vi "_FPGA System Polling.vi"(4 "error in (no error)":errorcluster, 5 "Waiting (F)":bool, 6 "Connected?":bool, 7 "CurInstrState":T3, 8 "High Vac Reached?":bool) -> (1 "Running":bool, 3 "Next InstrState":T3)   [LabVIEW 2018]
uses:
  Type/_RT Instrument State.ctl
  Type/_RT Polling Settings.ctl
  Type/_LCD Line2 Msg.ctl
  Type/_LED States.ctl
  Type/_LCD Line1 Msg.ctl
  Type/_RW Status.ctl
  Type/_Pump Parameter.ctl
  _RT Global.vi
  <vilib>/Utility/error.llb/Error Cluster From Error Code.vi
  <vilib>/rvi/errors/niLvFpgaAdjustHostInterfaceError.vi
  <vilib>/rvi/interface/nirviReadWriteControl/nirviReadWriteControl.xnode
  Type/FPGA Typedef.ctl
  FPGA Bitfiles/FPGA9607.lvbitx
  NiFpgaLv.dll
panel:
  out "Raw Reading":sgl
  in  "Polling Settings":T1[](array[typedef])=[{"ADC Ch"=119, "UserVal"=FALSE, "LowVal"=0.0, "HighVal"=89.0, "Fail Level"=50, "Err"="VG Disconnected/Broken Warning", "Line2Msg"=13, "InstrState"=enum."Ready", "Code"="004"}, {"ADC Ch"=119, "UserVal"=FALSE, "LowVal"=255.0, "HighVal"=300.0, "Fail Level"=50, "Err"="VG Disconnected/Broken Warning", "Line2Msg"=13, "InstrState"=enum."Ready", "Code"="004"}, {"ADC Ch"=119, "UserVal"=FALSE, "LowVal"=150.0, "HighVal"=254.0, "Fail Level"=50, "Err"="Overpressure Warning", "Line2Msg"=13, "InstrState"=enum."Ready", "Code"="006"}, {"ADC Ch"=64, "UserVal"=FALSE, "LowVal"=-5.0, "HighVal"=0.249, "Fail Level"=39, "Err"="Drying Gas Low", "Line2Msg"=4, "InstrState"=enum."Turbopump Ready", "Code"=""}, {"ADC Ch"=74, "UserVal"=FALSE, "LowVal"=0.36, "HighVal"=5.0, "Fail Level"=10, "Err"="Foreline Pressure Failure", "Line2Msg"=2, "InstrState"=enum."Fault", "Code"="001"}, {"ADC Ch"=25, "UserVal"=TRUE, "LowVal"=91.0, "HighVal"=200.0, "Fail Level"=35, "Err"="Q2 Board Slot 5 Overheating", "Line2Msg"=5, "InstrState"=enum."Turbopump Ready-Waiting", "Code"="008"}, {"ADC Ch"=49, "UserVal"=TRUE, "LowVal"=91.0, "HighVal"=200.0, "Fail Level"=35, "Err"="Q1 Board Slot 9 Overheating", "Line2Msg"=5, "InstrState"=enum."Turbopump Ready-Waiting", "Code"="009"}, {"ADC Ch"=57, "UserVal"=TRUE, "LowVal"=91.0, "HighVal"=200.0, "Fail Level"=35, "Err"="M1RF Board Slot 13 Overheating", "Line2Msg"=5, "InstrState"=enum."Turbopump Ready-Waiting", "Code"="010"}, {"ADC Ch"=26, "UserVal"=TRUE, "LowVal"=91.0, "HighVal"=200.0, "Fail Level"=35, "Err"="Q2 Board Slot 5 Overheating", "Line2Msg"=5, "InstrState"=enum."Turbopump Ready-Waiting", "Code"="008"}, {"ADC Ch"=50, "UserVal"=TRUE, "LowVal"=91.0, "HighVal"=200.0, "Fail Level"=35, "Err"="Q1 Board Slot 9 Overheating", "Line2Msg"=5, "InstrState"=enum."Turbopump Ready-Waiting", "Code"="009"}, {"ADC Ch"=58, "UserVal"=TRUE, "LowVal"=91.0, "HighVal"=200.0, "Fail Level"=35, "Err"="M1RF Board Slot 13 Overheating", "Line2Msg"=5, "InstrState"=enum."Turbopump Ready-Waiting", "Code"="010"}, {"ADC Ch"=113, "UserVal"=FALSE, "LowVal"=1.0, "HighVal"=2.0, "Fail Level"=40, "Err"="Source 1 Interlock Activated", "Line2Msg"=6, "InstrState"=enum."Source Standby", "Code"=""}, {"ADC Ch"=114, "UserVal"=FALSE, "LowVal"=1.0, "HighVal"=2.0, "Fail Level"=40, "Err"="Source 2 Interlock Activated", "Line2Msg"=7, "InstrState"=enum."Source Standby", "Code"=""}, {"ADC Ch"=14, "UserVal"=FALSE, "LowVal"=4.5, "HighVal"=10.0, "Fail Level"=35, "Err"="Heater PS Current High", "Line2Msg"=8, "InstrState"=enum."Turbopump Ready-Waiting", "Code"="011"}, {"ADC Ch"=51, "UserVal"=TRUE, "LowVal"=-9999.0, "HighVal"=-12.0, "Fail Level"=35, "Err"="Q1 Tuning Error", "Line2Msg"=5, "InstrState"=enum."Turbopump Ready-Waiting", "Code"="012"}, {"ADC Ch"=27, "UserVal"=TRUE, "LowVal"=-9999.0, "HighVal"=-12.0, "Fail Level"=35, "Err"="Q2 Tuning Error", "Line2Msg"=5, "InstrState"=enum."Turbopump Ready-Waiting", "Code"="013"}, {"ADC Ch"=59, "UserVal"=TRUE, "LowVal"=-9999.0, "HighVal"=-12.0, "Fail Level"=35, "Err"="M1 Tuning Error", "Line2Msg"=5, "InstrState"=enum."Turbopump Ready-Waiting", "Code"="014"}, {"ADC Ch"=120, "UserVal"=FALSE, "LowVal"=0.0, "HighVal"=0.0, "Fail Level"=32, "Err"="Card Cage Door Interlock Activated", "Line2Msg"=9, "InstrState"=enum."Go to 24V Standby", "Code"=""}, {"ADC Ch"=121, "UserVal"=FALSE, "LowVal"=0.0, "HighVal"=0.0, "Fail Level"=35, "Err"="Vacuum Ready Tripped", "Line2Msg"=2, "InstrState"=enum."Turbopump Ready-Waiting", "Code"="015"}, {"ADC Ch"=76, "UserVal"=FALSE, "LowVal"=0.0, "HighVal"=2.5, "Fail Level"=39, "Err"="Drying Gas Supply Low", "Line2Msg"=4, "InstrState"=enum."Turbopump Ready", "Code"=""}, {"ADC Ch"=78, "UserVal"=FALSE, "LowVal"=0.0, "HighVal"=3.5, "Fail Level"=39, "Err"="Source Gas Supply Low", "Line2Msg"=12, "InstrState"=enum."Turbopump Ready", "Code"=""}, {"ADC Ch"=100, "UserVal"=FALSE, "LowVal"=0.0, "HighVal"=0.0, "Fail Level"=32, "Err"="Electronics is off", "Line2Msg"=5, "InstrState"=enum."Go to 24V Standby", "Code"="017"}, {"ADC Ch"=72, "UserVal"=FALSE, "LowVal"=-1.0, "HighVal"=0.3, "Fail Level"=49, "Err"="Exhaust Gas Low", "Line2Msg"=15, "InstrState"=enum."Ready", "Code"=""}, {"ADC Ch"=81, "UserVal"=TRUE, "LowVal"=26.0, "HighVal"=30.0, "Fail Level"=50, "Err"="RF Board Power Supply Error", "Line2Msg"=0, "InstrState"=enum."Ready", "Code"=""}, {"ADC Ch"=82, "UserVal"=TRUE, "LowVal"=-30.0, "HighVal"=-26.0, "Fail Level"=50, "Err"="RF Board Power Supply Error", "Line2Msg"=0, "InstrState"=enum."Ready", "Code"=""}, {"ADC Ch"=83, "UserVal"=TRUE, "LowVal"=45.0, "HighVal"=65.0, "Fail Level"=50, "Err"="Heater Power Supply Error", "Line2Msg"=0, "InstrState"=enum."Ready", "Code"=""}, {"ADC Ch"=85, "UserVal"=TRUE, "LowVal"=22.0, "HighVal"=26.0, "Fail Level"=50, "Err"="24 V Mains Power Supply Error", "Line2Msg"=0, "InstrState"=enum."Ready", "Code"=""}, {"ADC Ch"=86, "UserVal"=TRUE, "LowVal"=13.0, "HighVal"=16.0, "Fail Level"=50, "Err"="ADC/Board Power Supply Error", "Line2Msg"=0, "InstrState"=enum."Ready", "Code"=""}, {"ADC Ch"=87, "UserVal"=TRUE, "LowVal"=-16.0, "HighVal"=-13.0, "Fail Level"=50, "Err"="ADC/Board Power Supply Error", "Line2Msg"=0, "InstrState"=enum."Ready", "Code"=""}] {"Line2Msg" items=["Same", "Empty", "VacFail", "Cancel", "CheckGas", "EleFail", "Probe1Fail", "Probe2Fail", "HeaterFail", "DoorOpen", "CheckComm", "PressStart", "CheckSource", "VacWarn", "ForelineHigh", "SourceExhaustLow"]}
  # "0   119  50 vacuum gauge disconnected\n1   119  50 vacuum gauge disconnected\n2   119  50 overpressure warning\n3   64    39 drying gas low\n4   74    10 foreline pressure failure\n5   25    35 Q2 board slot 5 overheating\n6   49    35 Q1 board slot 9 overheating\n7   57    35 M1RF board slot 13 overheating\n8   26    35 Q2 board slot 5 overheating\n9   50    35 Q1 board slot 9 overheating\n10  58    35 M1RF board slot 13 overheating\n11 113  40 source 1 interlock activated\n12 114  40 source 2 interlock activated\n13  14    35 heater PS currect high\n14  51    35 Q1 tuning error\n15  27    35 Q2 tuning error\n16  59    35 M1 tuning error\n17 120  32 card cage door interlock activated\n18 121  35 vacuum ready tripped\n19  76    40 drying gas supply low\n20  78    40 source gas supply low\n21 100  32 electronics is off\n22  72    50 exhaust gas low\n23  81    50 RF board power supply error\n24  82    50 RF board power supply error\n25  83    50 heater power supply error\n26  85    50 24 V mains power supply error\n27  86    50 ADC/board power supply error\n28  87    50 ADC/board power supply error"
  # "same"
  # "4.6 -> 5.1"
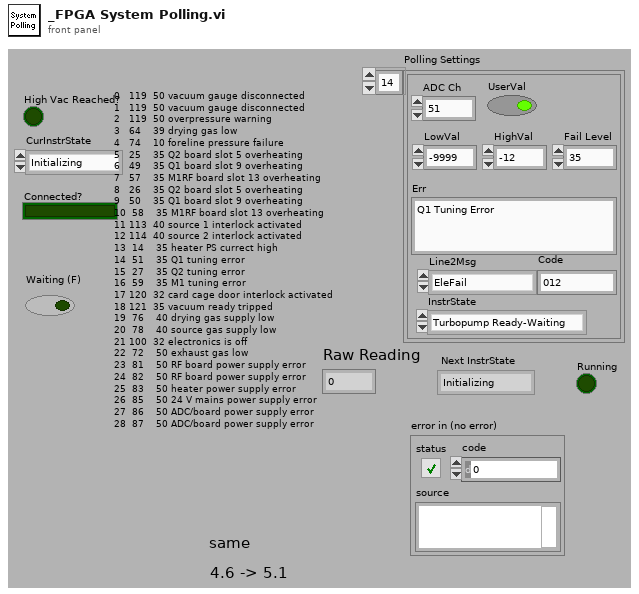
[diagram p1: front panel]
types:
  T1 = typedef "_RT Polling Settings.ctl" = cluster{"ADC Ch":u8, "UserVal":bool, "LowVal":sgl, "HighVal":sgl, "Fail Level":u8, "Err":string, "Line2Msg":T2, "InstrState":T3, "Code":string}
  T2 = typedef "_LCD Line2 Msg.ctl" = u16
  T3 = typedef "_RT Instrument State.ctl" = enum16{"Initializing", "Mass Spectrometer is Off", "Starting Up", "Turning Power Off", "Going to Standby", "Roughing Pump Ready", "Turning Turbo Off", "Turbo Startup", "Turbopump Ready", "Checking Vacuum", "Going to Ready", "Ready", "Running", "Source Standby", "Lost Communication", "Shutting Down", "Fault", "24V Standby", "Go to 24V Standby", "Turbopump Ready-Waiting"}
  T4 = typedef "_RT Startup Options.ctl" = cluster{"Door":bool, "Curtain":bool, "Pressure":bool, "Turbo":bool, "SysPoll":bool, "GasFlag":bool, "SourceExhaust":bool}
  T5 = typedef "_LED States.ctl" = enum8{"Idle", "Solid B", "Solid R", "Solid P", "Off B", "Off R", "Off P", "Off BRP", "Off RP", "Flash R&P", "Flash P"}
  T6 = typedef "_Pump Parameter.ctl" = enum16{"Turn Pump Motor On", "Turn Pump Motor Off", "Read Pump Oil Deficiency", "Read Rotation Switch Point Attained", "Read Ele. Drive Over Temperature", "Read Pump Over Temperature", "Read Set Rotation Speed Attained", "Read Turbopump Accelerates", "Read Actual Rotation Speed in Hz", "Read Motor Current in A", "Read Operating Hours in h", "Read Motor Voltage in V", "Read Motor Power in W", "Set Rotation Speed Switchpoint in %", "Clear Error", "Read Error Code", "Read Bearing Temperature", "Read Hardware Version", "Read Firmware Version", "Read Operating Hours (Drive)", "Read Rotational Speed (rpm)", "Read Power Stage Temperature", "Read Electronics Temperature", "Read Upper Pump Temperature", "Read Motor Temperature", "Read Error Code History, 1", "Read Error Code History, 2", "Read Error Code History, 3", "Read Error Code History, 4", "Read Error Code History, 5", "Read Error Code History, 6", "Read Error Code History, 7", "Read Error Code History, 8", "Read Error Code History, 9", "Read Error Code History, 10"}
  T7 = typedef "_RW Status.ctl" = enum8{"Done", "Do Read", "Do Write", "Set Latch1", "Set Latch2", "Set Latch3", "Set Latch4", "RP ON", "EL ON", "Serial Send", "Set LC Out", "Get LC In", "Read VAC", "Table Test", "Get Interlock", "Do Read2", "Do Write2"}
  T8 = typedef "FPGA Typedef.ctl" = refnum<k20>
  T9 = typedef "_LCD Line1 Msg.ctl" = u16
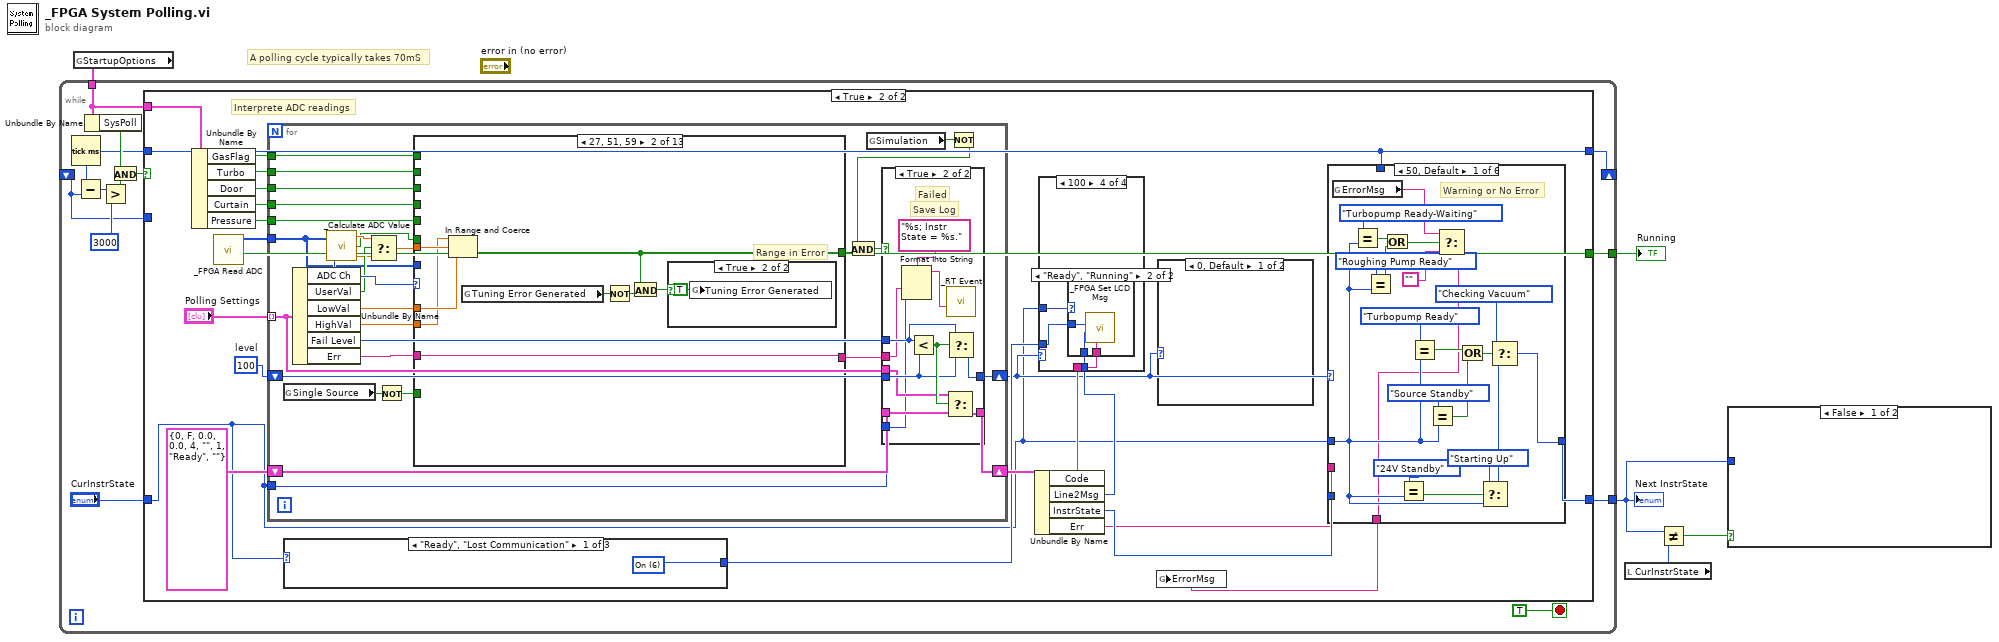
[diagram p0: block diagram]
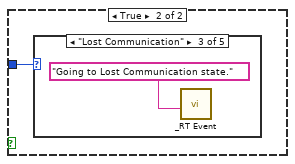
[diagram p2: hidden frame]
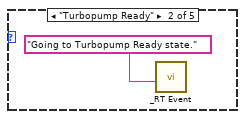
[diagram p4: hidden frame]
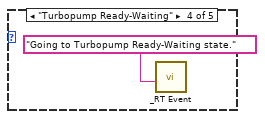
[diagram p5: hidden frame]
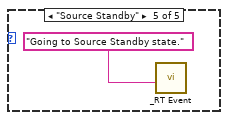
[diagram p6: hidden frame]
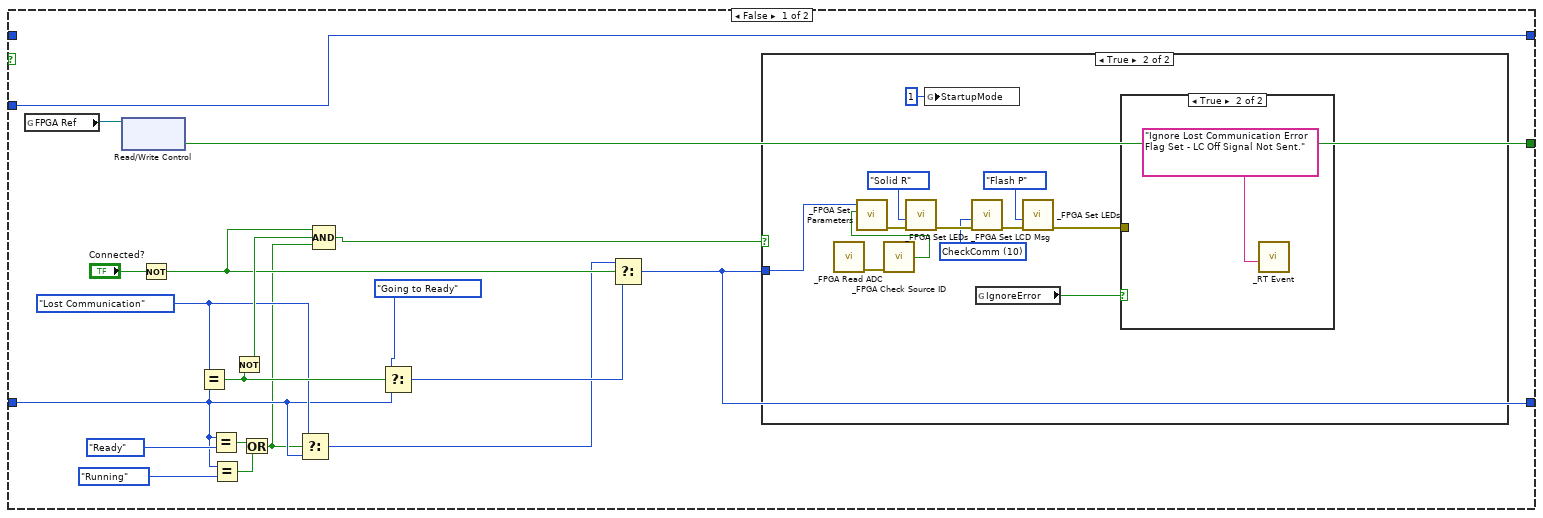
[diagram p7: hidden frame]
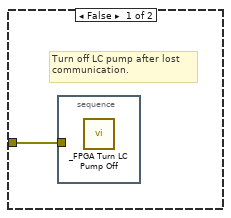
[diagram p9: hidden frame]
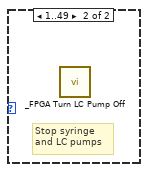
[diagram p10: hidden frame]
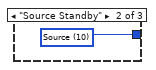
[diagram p11: hidden frame]
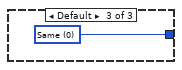
[diagram p12: hidden frame]
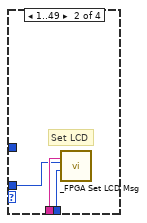
[diagram p14: hidden frame]
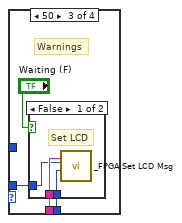
[diagram p15: hidden frame]
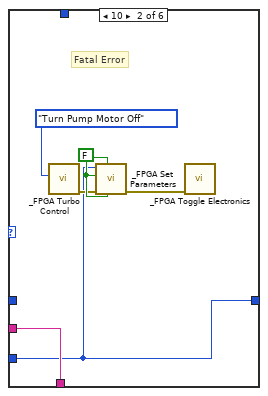
[diagram p18: hidden frame]
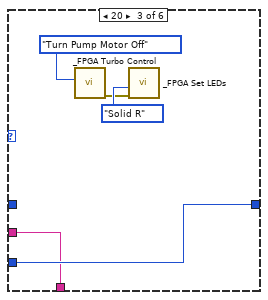
[diagram p19: hidden frame]
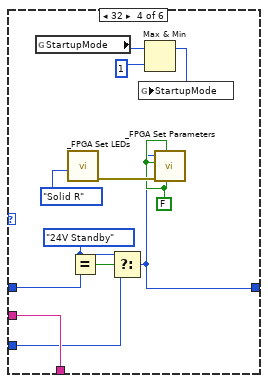
[diagram p20: hidden frame]
diagram:
  # "A polling cycle typically takes 70mS"
  n1 = global read "_RT Global.vi" "StartupOptions"() -> (w4:T4)
  n2 = while {
    tunnel: [w16] -> w1
    shift-right: [w7] -> _
    shift-left: _ -> [w6]
    tunnel: [w13] -> w5
    tunnel: w4 -> [w9]
    stop <- TRUE stop-if-true
    n3 = Tick Count (ms)() -> (millisecond timer value=w8:u32)
    n4 = Subtract(x=w8, y=w6) -> (x-y=w15:u32)
    n5 = Unbundle By Name(w9) -> ("SysPoll"=w12:bool)
    n6 = Greater?(x=w15, y=3000) -> (0:w11:bool)
    n7 = And(x=w12, y=w11) -> (x .and. y?=w10:bool)
    n8 = case shown="True" w10 {
      tunnel: [w19 w70] -> w16
      tunnel: "CurInstrState" -> [w24 w52]
      tunnel: [w30 w73] -> w13
      tunnel: w9 -> [_ w68]
      tunnel: w8 -> [_ w53]
      tunnel: [w33 w53] -> w7
      tunnel: w6 -> [w33 _]
      frame False {
        w25 = _RT_Instrument_State."Lost Communication" ("t")
        n9 = global read "_RT Global.vi" "FPGA Ref"() -> (w21:T8)
        n10 = xnode "Read/Write Control"("FPGA VI Reference In"=w21) -> ("Running"=w30:bool)  [unwired: 1 in, 2 out]
        n11 = Not(x="Connected?") -> (.not. x?=w32:bool)
        n12 = Equal?(x=w25, y=w24) -> (x = y?=w35:bool)
        n13 = Equal?(x=w24, y=_RT_Instrument_State."Ready") -> (x = y?=w27:bool)
        n14 = Equal?(x=w24, y=_RT_Instrument_State."Running") -> (x = y?=w26:bool)
        n15 = Not(x=w35) -> (.not. x?=w34:bool)
        n16 = Or(x=w27, y=w26) -> (x .or. y?=w22:bool)
        n17 = Select(t=w25, s=w22, f=w24) -> (s? t:f=w23:T3)
        n18 = Compound Arithmetic op=AND(w32, w34, w22) -> (w20:bool)
        n19 = Select(t=_RT_Instrument_State."Going to Ready", s=w35, f=w24) -> (s? t:f=w36:T3)
        n20 = Select(t=w23, s=w32, f=w36) -> (s? t:f=w19:T3)
        n21 = case shown="True" w20 {
          tunnel: w19 -> [_ w38]
          frame False {
          }
          frame True {
            w43 = T2 10 items=["Same", "Empty", "VacFail", "Cancel", "CheckGas", "EleFail", "Probe1Fail", "Probe2Fail", "HeaterFail", "DoorOpen", "CheckComm", "PressStart", "StartRP"] ("Line2Msg (same)")
            n22 = call "_FPGA Read ADC.vi"() -> ("error out"=w45:errorcluster)  [unwired: 3 in, 6 out]
            n23 = call "_FPGA Check Source ID.vi"("error in (no error)"=w45) -> ("Source ID OK"=w44:bool)
            n24 = call "_FPGA Set Parameters.vi"("HSID Temp (on)"=w44, "CurInstrState"=w38) -> ("error out"=w41:errorcluster)  [unwired: 7 in, 2 out]
            n25 = call "_FPGA Set LEDs.vi"("error in (no error)"=w41, "LED Command"=_LED_States."Solid R") -> ("error out"=w48:errorcluster)  [unwired: 2 in, 3 out]
            n26 = global write "_RT Global.vi" "StartupMode"(u8 1 ("StartupMode")) -> ()
            n27 = call "_FPGA Set LCD Msg.vi"("error in"=w48, "Line2Msg (same)"=w43) -> ("error out"=w46:errorcluster)  [unwired: 5 in, 2 out]
            n28 = global read "_RT Global.vi" "IgnoreError"() -> (w39:bool)
            n29 = call "_FPGA Set LEDs.vi"("error in (no error)"=w46, "LED Command"=_LED_States."Flash P") -> ("error out"=w40:errorcluster)  [unwired: 2 in, 3 out]
            n30 = case shown="True" w39 {
              tunnel: w40 -> [w50 _]
              frame False {
                # "Turn off LC pump after lost\ncommunication."
                n31 = stacked-sequence {
                  tunnel: w50 -> [_]
                  frame #0 {
                    n32 = call "_FPGA Turn LC Pump Off.vi"() -> ()  [unwired: 2 in]
                  }
                }
              }
              frame True {
                n33 = call "_RT Event.vi"("Event"="Ignore Lost Communication Error Flag Set - LC Off Signal Not Sent.") -> ()  [unwired: 2 in, 5 out]
              }
            }
          }
        }
      }
      frame True {
        w71 = u8 100  # level
        # "Interprete ADC readings"
        n34 = Unbundle By Name(w68) -> ("GasFlag"=w57:bool, "Turbo"=w64:bool, "Door"=w67:bool, "Curtain"=w66:bool, "Pressure"=w65:bool)
        n35 = call "_FPGA Read ADC.vi"() -> ("Running"=w73:bool, "ADC Values"=w72:i32[])  [unwired: 3 in, 5 out]
        n36 = for {
          tunnel: w72 -> [w159]
          shift-right: [w175] -> w56
          shift-left: w71 -> [w177]
          tunnel: "Polling Settings" -> [w166] mode=indexing
          shift-right: [w174] -> w62
          shift-left: T1 {"ADC Ch"=0, "UserVal"=FALSE, "LowVal"=0.0, "HighVal"=0.0, "Fail Level"=4, "Err"="", "Line2Msg"=1, "InstrState"=enum."Ready", "Code"=""} ("Cluster") -> [w176]
          tunnel: w67 -> [w170]
          tunnel: w66 -> [w169]
          tunnel: w65 -> [w168]
          tunnel: w64 -> [w167]
          tunnel: w57 -> [w165]
          tunnel: w52 -> [w155]
          n37 = global read "_RT Global.vi" "Single Source"() -> (w164:bool)
          n38 = Unbundle By Name(w166) -> ("ADC Ch"=w183:u8, "UserVal"=w182:bool, "LowVal"=w179:sgl, "HighVal"=w178:sgl, "Fail Level"=w173:u8, "Err"=w157:string)
          n39 = call "_Calculate ADC Value.vi"("ADC Values"=w159, "ADC Channel (64)"=w183) -> ("User Value"=w181:sgl, "In Range?"=w158:bool, "Raw Reading"=w180:sgl)
          n40 = Select(t=w181, s=w182, f=w180) -> (s? t:f=w171:sgl)
          n41 = Not(x=w164) -> (.not. x?=w163:bool)
          n42 = case shown="27, 51, 59" w183 {
            selector: w183 -> [_ _ _ _ w226 _ w262 _ w302 w319 _ _ _]
            tunnel: w171 -> [w201 w209 w216 w221 w232 w257 _ w286 _ _ _ _ _]
            tunnel: w179 -> [w200 w208 w215 _ w228 w256 _ w281 _ _ _ _ _]
            tunnel: w178 -> [w199 w207 w214 _ w229 w255 _ w280 _ _ _ _ _]
            tunnel: [w198 w204 w212 w217 w227 w253 w263 w282 w303 w321 w341 FALSE w382] -> w172
            tunnel: w170 -> [_ _ _ _ _ _ _ _ _ _ w343 _ _]
            tunnel: w169 -> [_ _ _ _ w225 _ _ _ _ _ _ _ _]
            tunnel: w168 -> [_ _ _ _ _ w252 _ _ _ _ _ _ _]
            tunnel: w167 -> [_ _ _ _ _ _ _ w284 _ _ _ _ _]
            tunnel: w165 -> [_ _ _ _ _ _ w261 _ _ _ _ _ _]
            tunnel: w163 -> [_ _ _ _ _ _ _ _ _ w318 _ _ _]
            tunnel: w159 -> [_ _ _ _ _ _ _ _ _ _ _ w372 _]
            tunnel: w158 -> [_ _ _ w223 _ _ w260 _ w305 w322 w340 _ w383]
            tunnel: w157 -> [w197 w206 w211 w222 w224 w251 w258 w279 w301 w317 w338 w348 w380]
            tunnel: [w197 w206 w211 w222 w224 w251 w258 w279 w301 w317 w338 w348 w379] -> w156
            frame Default {
              # "Range in Error"
              n43 = In Range and Coerce(upper limit=w199, x=w201, lower limit=w200) -> (In Range?=w198:bool)  [unwired: 1 out]
            }
            frame 27, 51, 59 {
              # "Range in Error"
              n44 = In Range and Coerce(upper limit=w207, x=w209, lower limit=w208) -> (In Range?=w204:bool)  [unwired: 1 out]
              n45 = global read "_RT Global.vi" "Tuning Error Generated"() -> (w205:bool)
              n46 = Not(x=w205) -> (.not. x?=w203:bool)
              n47 = And(x=w204, y=w203) -> (x .and. y?=w202:bool)
              n48 = case shown="True" w202 {
                frame False {
                }
                frame True {
                  n49 = global write "_RT Global.vi" "Tuning Error Generated"(TRUE ("Tuning Error Generated")) -> ()
                }
              }
            }
            frame 20..23, 81..97 {
              # "Allowable Range"
              n50 = In Range and Coerce(upper limit=w214, x=w216, lower limit=w215) -> (In Range?=w213:bool)  [unwired: 1 out]
              n51 = Not(x=w213) -> (.not. x?=w212:bool)
            }
            frame 72 {
              # "Check for exhaust gas"
              n52 = Not(x=w223) -> (.not. x?=w218:bool)
              n53 = global write "_RT Global.vi" "Exhaust gas error"(w218) -> ()
              n54 = global read "_RT Global.vi" "Tuning Error Generated"() -> (w220:bool)
              n55 = Not(x=w220) -> (.not. x?=w219:bool)
              n56 = And(x=w218, y=w219) -> (x .and. y?=w217:bool)
              "Raw Reading" <- w221
            }
            frame 64 {
              # "Curtain Gas"
              n57 = In Range and Coerce(upper limit=w229, x=w232, lower limit=w228) -> (In Range?=w231:bool)  [unwired: 1 out]
              n58 = And(x=w225, y=w231) -> (x .and. y?=w230:bool)
              n59 = case shown="True" w230 {
                selector: w230 -> [w233 _]
                tunnel: [w233 w238] -> w227
                tunnel: w228 -> [_ w237]
                tunnel: w229 -> [_ w236]
                tunnel: w226 -> [_ w235]
                tunnel: w225 -> [_ w234]
                frame False {
                }
                frame True {
                  n60 = while {
                    tunnel: [w239] -> w238
                    tunnel: w237 -> [w250]
                    tunnel: w236 -> [w249]
                    tunnel: w235 -> [w243]
                    tunnel: w234 -> [w242]
                    i -> [w248]
                    stop <- w246 continue-if-true
                    n61 = call "_FPGA Read ADC.vi"("ADC Channel (64)"=w243) -> ("Raw Reading"=w244:sgl)  [unwired: 2 in, 6 out]
                    n62 = In Range and Coerce(upper limit=w249, x=w244, lower limit=w250) -> (In Range?=w241:bool)  [unwired: 1 out]
                    n63 = Less?(x=w248, y=2) -> (x < y?=w240:bool)
                    n64 = Wait (ms)(milliseconds to wait=u32 280) -> ()  [unwired: 1 out]
                    n65 = And(x=w242, y=w241) -> (x .and. y?=w239:bool)
                    n66 = And(x=w239, y=w240) -> (x .and. y?=w246:bool)
                  }
                }
              }
            }
            frame 74 {
              # "Foreline Pressure"
              n67 = In Range and Coerce(upper limit=w255, x=w257, lower limit=w256) -> (In Range?=w254:bool)  [unwired: 1 out]
              n68 = And(x=w252, y=w254) -> (x .and. y?=w253:bool)
            }
            frame 76, 78 {
              # "For Auto Gas Flags"
              n69 = Not(x=w260) -> (.not. x?=w259:bool)
              n70 = And(x=w261, y=w259) -> (x .and. y?=w264:bool)
              n71 = case shown="True" w264 {
                selector: w264 -> [w265 _]
                tunnel: [w265 w268] -> w263
                tunnel: w262 -> [_ w267]
                tunnel: w261 -> [_ w266]
                frame False {
                }
                frame True {
                  n72 = while {
                    tunnel: [w271] -> w268
                    tunnel: w267 -> [w274]
                    tunnel: w266 -> [w273]
                    i -> [w278]
                    stop <- w276 continue-if-true
                    n73 = call "_FPGA Read ADC.vi"("ADC Channel (64)"=w274) -> ("In Range?"=w270:bool)  [unwired: 2 in, 6 out]
                    n74 = Not(x=w270) -> (.not. x?=w269:bool)
                    n75 = Less?(x=w278, y=2) -> (x < y?=w272:bool)
                    n76 = Wait (ms)(milliseconds to wait=u32 280) -> ()  [unwired: 1 out]
                    n77 = And(x=w273, y=w269) -> (x .and. y?=w271:bool)
                    n78 = And(x=w271, y=w272) -> (x .and. y?=w276:bool)
                  }
                }
              }
            }
            frame 119 {
              # "High Pressure"
              n79 = In Range and Coerce(upper limit=w280, x=w286, lower limit=w281) -> (In Range?=w285:bool)  [unwired: 1 out]
              n80 = And(x=w284, y=w285) -> (x .and. y?=w283:bool)
              n81 = case shown="False" w283 {
                selector: w283 -> [w287 _]
                tunnel: [w287 w290] -> w282
                tunnel: w281 -> [_ w289]
                tunnel: w280 -> [_ w288]
                frame False {
                }
                frame True {
                  n82 = while {
                    tunnel: [w294] -> w290
                    tunnel: w289 -> [w300]
                    tunnel: w288 -> [w299]
                    i -> [w296]
                    stop <- w292 continue-if-true
                    n83 = call "_FPGA Read Data.vi"("Read Mode (Do Read)"=_RW_Status."Read VAC" ("R/W Status")) -> ("Data"=w297:u32)  [unwired: 4 in, 2 out]
                    n84 = In Range and Coerce(upper limit=w299, x=w297, lower limit=w300) -> (In Range?=w294:bool)  [unwired: 1 out]
                    n85 = Less?(x=w296, y=4) -> (x < y?=w293:bool)
                    n86 = Wait (ms)(milliseconds to wait=u32 180) -> ()  [unwired: 1 out]
                    n87 = And(x=w293, y=w294) -> (x .and. y?=w292:bool)
                  }
                }
              }
            }
            frame 113 {
              # "for source ID 1"
              n88 = Not(x=w305) -> (.not. x?=w304:bool)
              n89 = case shown="True" w304 {
                selector: w304 -> [w306 _]
                tunnel: [w306 w308] -> w303
                tunnel: w302 -> [_ w307]
                frame False {
                }
                frame True {
                  n90 = while {
                    tunnel: [w309] -> w308
                    tunnel: w307 -> [w311]
                    i -> [w316]
                    stop <- w313 continue-if-true
                    n91 = call "_FPGA Read ADC.vi"("ADC Channel (64)"=w311) -> ("In Range?"=w310:bool)  [unwired: 2 in, 6 out]
                    n92 = Not(x=w310) -> (.not. x?=w309:bool)
                    n93 = Wait (ms)(milliseconds to wait=u32 280) -> ()  [unwired: 1 out]
                    n94 = Less?(x=w316, y=2) -> (x < y?=w314:bool)
                    n95 = And(x=w314, y=w309) -> (x .and. y?=w313:bool)
                  }
                }
              }
            }
            frame 114 {
              # "for source ID 2"
              n96 = Not(x=w322) -> (.not. x?=w323:bool)
              n97 = And(x=w323, y=w318) -> (x .and. y?=w320:bool)
              n98 = case shown="False" w320 {
                selector: w320 -> [w324 _]
                tunnel: [w324 w327] -> w321
                tunnel: w319 -> [_ w326]
                tunnel: w318 -> [_ w325]
                frame False {
                }
                frame True {
                  n99 = while {
                    tunnel: [w328] -> w327
                    tunnel: w326 -> [w332]
                    tunnel: w325 -> [w330]
                    i -> [w337]
                    stop <- w334 continue-if-true
                    n100 = call "_FPGA Read ADC.vi"("ADC Channel (64)"=w332) -> ("In Range?"=w331:bool)  [unwired: 2 in, 6 out]
                    n101 = Not(x=w331) -> (.not. x?=w329:bool)
                    n102 = Wait (ms)(milliseconds to wait=u32 280) -> ()  [unwired: 1 out]
                    n103 = And(x=w329, y=w330) -> (x .and. y?=w328:bool)
                    n104 = Less?(x=w337, y=2) -> (x < y?=w335:bool)
                    n105 = And(x=w335, y=w328) -> (x .and. y?=w334:bool)
                  }
                }
              }
            }
            frame 120 {
              # "for door interlock"
              n106 = Not(x=w340) -> (.not. x?=w339:bool)
              n107 = And(x=w343, y=w339) -> (x .and. y?=w342:bool)
              n108 = case shown="True" w342 {
                selector: w342 -> [w344 _]
                tunnel: [w344 w345] -> w341
                frame False {
                }
                frame True {
                  # "if fail, do a direct read"
                  n109 = call "_FPGA Read Data.vi"("Read Mode (Do Read)"=_RW_Status."Get Interlock" ("R/W Status")) -> ("Data"=w346:u32)  [unwired: 4 in, 2 out]
                  n110 = Equal To 0?(x=w346) -> (x = 0?=w345:bool)
                }
              }
            }
            frame 100 {
              w350 = sgl 0.5 ("y")
              # "Check for electronics off"
              n111 = global read "_RT Global.vi" "Ele On"() -> (w358:bool)
              n112 = call "_Calculate ADC Value.vi"("ADC Values"=w372, "ADC Channel (64)"=u8 20) -> ("Raw Reading"=w371:sgl)  [unwired: 2 out]
              n113 = call "_Calculate ADC Value.vi"("ADC Values"=w372, "ADC Channel (64)"=u8 21) -> ("Raw Reading"=w369:sgl)  [unwired: 2 out]
              n114 = call "_Calculate ADC Value.vi"("ADC Values"=w372, "ADC Channel (64)"=u8 88) -> ("Raw Reading"=w368:sgl)  [unwired: 2 out]
              n115 = call "_Calculate ADC Value.vi"("ADC Values"=w372, "ADC Channel (64)"=u8 89) -> ("Raw Reading"=w367:sgl)  [unwired: 2 out]
              n116 = call "_Calculate ADC Value.vi"("ADC Values"=w372, "ADC Channel (64)"=u8 96) -> ("Raw Reading"=w366:sgl)  [unwired: 2 out]
              n117 = call "_Calculate ADC Value.vi"("ADC Values"=w372, "ADC Channel (64)"=u8 97) -> ("Raw Reading"=w370:sgl)  [unwired: 2 out]
              n118 = Absolute Value(x=w370) -> (abs(x)=w351:sgl)
              n119 = Absolute Value(x=w369) -> (abs(x)=w355:sgl)
              n120 = Absolute Value(x=w366) -> (abs(x)=w352:sgl)
              n121 = Absolute Value(x=w371) -> (abs(x)=w356:sgl)
              n122 = Absolute Value(x=w367) -> (abs(x)=w353:sgl)
              n123 = Absolute Value(x=w368) -> (abs(x)=w354:sgl)
              n124 = Not(x=w358) -> (.not. x?=w359:bool)
              n125 = Less?(x=w356, y=w350) -> (x < y?=w365:bool)
              n126 = Less?(x=w355, y=w350) -> (x < y?=w362:bool)
              n127 = Less?(x=w354, y=w350) -> (x < y?=w363:bool)
              n128 = Less?(x=w353, y=w350) -> (x < y?=w361:bool)
              n129 = Less?(x=w352, y=w350) -> (x < y?=w360:bool)
              n130 = Less?(x=w351, y=w350) -> (x < y?=w364:bool)
              n131 = Compound Arithmetic op=AND(w365, w362, w363, w361, w360, w364) -> (w357:bool)
              n132 = Or(x=w359, y=w357) -> ()  [unwired: 1 out]
            }
            frame 121 {
              # "for vacuum ready interlock"
              n133 = Not(x=w383) -> (.not. x?=w382:bool)
              n134 = case shown="False" "High Vac Reached?" {
                tunnel: [w384 "High Vacuum Not Achieved" ("Err")] -> w379
                tunnel: w380 -> [w384 _]
                frame True {
                }
                frame False {
                }
              }
            }
          }
          n135 = global read "_RT Global.vi" "Simulation"() -> (w162:bool)
          n136 = Not(x=w162) -> (.not. x?=w160:bool)
          n137 = And(x=w160, y=w172) -> (x .and. y?=w161:bool)
          n138 = case shown="True" w161 {
            tunnel: w177 -> [w185 w194]
            tunnel: [w185 w193] -> w175
            tunnel: w173 -> [_ w195]
            tunnel: w176 -> [w184 w190]
            tunnel: [w184 w192] -> w174
            tunnel: w156 -> [_ w188]
            tunnel: w166 -> [_ w191]
            tunnel: w155 -> [_ w187]
            frame False {
              # "Passed"
            }
            frame True {
              # "Save Log"
              # "Failed"
              n139 = Format Into String(format string="%s; Instr State = %s.", w188, w187) -> (resulting string=w186:string)  [unwired: 2 in, 1 out]
              n140 = Less?(x=w195, y=w194) -> (x < y?=w196:bool)
              n141 = Select(t=w191, s=w196, f=w190) -> (s? t:f=w192:T1)
              n142 = call "_RT Event.vi"("Event"=w186) -> ()  [unwired: 2 in, 5 out]
              n143 = Select(t=w195, s=w196, f=w194) -> (s? t:f=w193:u8)
            }
          }
        }
        n144 = case shown="\"Ready\", \"Lost Communication\"" w52 {
          tunnel: [w74 w75 w76] -> w58
          frame "Ready", "Lost Communication" {
            w74 = T9 6 items=["Same", "Empty", "Connected", "Starting", "Stopping", "Action", "On", "Service", "Call", "Acquiring", "Source"] ("Line1Msg (same)")
          }
          frame "Source Standby" {
            w75 = T9 10 items=["Same", "Empty", "Connected", "Starting", "Stopping", "Action", "On", "Service", "Call", "Acquiring", "Source"] ("Line1Msg (same)")
          }
          frame Default {
            w76 = T9 0 items=["Same", "Empty", "Connected", "Starting", "Stopping", "Action", "On", "Service", "Call", "Acquiring", "Source"] ("Line1Msg (same)")
          }
        }
        n145 = Unbundle By Name(w62) -> ("Code"=w59:string, "Line2Msg"=w60:T2, "InstrState"=w61:T3, "Err"=w55:string)
        n146 = case shown="100" w56 {
          tunnel: w60 -> [_ w79 w83 w89]
          tunnel: w59 -> [_ w78 w82 w88]
          tunnel: w58 -> [_ w77 w81 w90]
          tunnel: w52 -> [_ _ _ w87]
          frame Default {
          }
          frame 1..49 {
            # "Set LCD"
            n147 = call "_FPGA Set LCD Msg.vi"("ErrNum"=w78, "Line2Msg (same)"=w79, "Line1Msg (same)"=w77) -> ()  [unwired: 4 in, 3 out]
          }
          frame 50 {
            # "Warnings"
            n148 = case shown="False" "Waiting (F)" {
              tunnel: w83 -> [w86 _]
              tunnel: w82 -> [w85 _]
              tunnel: w81 -> [w84 _]
              frame False {
                # "Set LCD"
                n149 = call "_FPGA Set LCD Msg.vi"("ErrNum"=w85, "Line2Msg (same)"=w86, "Line1Msg (same)"=w84) -> ()  [unwired: 4 in, 3 out]
              }
              frame True {
              }
            }
          }
          frame 100 {
            n150 = case shown="\"Ready\", \"Running\"" w87 {
              tunnel: w90 -> [_ w93]
              tunnel: w89 -> [_ w92]
              tunnel: w88 -> [_ w91]
              frame Default {
              }
              frame "Ready", "Running" {
                n151 = call "_FPGA Set LCD Msg.vi"("ErrNum"=w91, "Line2Msg (same)"=w92, "Line1Msg (same)"=w93) -> ()  [unwired: 4 in, 3 out]
              }
            }
          }
        }
        n152 = case shown="0, Default" w56 {
          frame 0, Default {
          }
          frame 1..49 {
            # "Stop syringe \nand LC pumps"
            n153 = call "_FPGA Turn LC Pump Off.vi"() -> ()  [unwired: 2 in]
          }
        }
        n154 = case shown="50, Default" w56 {
          tunnel: w52 -> [w100 _ _ w132 _ _]
          tunnel: [w107 w114 w122 w125 w137 w146] -> w70
          tunnel: w61 -> [_ w114 w122 w129 w137 w146]
          tunnel: w55 -> [_ w117 w121 w133 w141 w151]
          tunnel: [w94 w117 w121 w133 w141 w151] -> w54
          tunnel: w53 -> [_ _ _ _ _ _]
          frame 50, Default {
            # "Warning or No Error"
            n155 = global read "_RT Global.vi" "ErrorMsg"() -> (w96:string)
            n156 = Equal?(x=_RT_Instrument_State."Turbopump Ready-Waiting", y=w100) -> (x = y?=w99:bool)
            n157 = Equal?(x=_RT_Instrument_State."Roughing Pump Ready", y=w100) -> (x = y?=w98:bool)
            n158 = Or(x=w99, y=w98) -> (x .or. y?=w97:bool)
            n159 = Equal?(x=_RT_Instrument_State."24V Standby", y=w100) -> (x = y?=w103:bool)
            n160 = Equal?(x=_RT_Instrument_State."Turbopump Ready", y=w100) -> (x = y?=w111:bool)
            n161 = Equal?(x=_RT_Instrument_State."Source Standby", y=w100) -> (x = y?=w110:bool)
            n162 = Select(t=w96, s=w97, f="") -> (s? t:f=w94:string)
            n163 = Or(x=w111, y=w110) -> (x .or. y?=w109:bool)
            n164 = Select(t=_RT_Instrument_State."Starting Up" ("x"), s=w103, f=w100) -> (s? t:f=w104:T3)
            n165 = Select(t=_RT_Instrument_State."Checking Vacuum" ("x"), s=w109, f=w104) -> (s? t:f=w107:T3)
          }
          frame 10 {
            w118 = FALSE
            # "Fatal Error"
            n166 = call "_FPGA Turbo Control.vi"("Command"=_Pump_Parameter."Turn Pump Motor Off") -> ("error out"=w116:errorcluster)  [unwired: 3 in, 5 out]
            n167 = call "_FPGA Set Parameters.vi"("ExhaustGas (on)"=w118, "CurGas (on)"=w118, "error in"=w116, "HSID Temp (on)"=w118, "CurInstrState"=w114) -> ("error out"=w115:errorcluster)  [unwired: 4 in, 2 out]
            n168 = call "_FPGA Toggle Electronics.vi"("error in"=w115) -> ()  [unwired: 2 in, 6 out]
          }
          frame 20 {
            n169 = call "_FPGA Turbo Control.vi"("Command"=_Pump_Parameter."Turn Pump Motor Off") -> ("error out"=w120:errorcluster)  [unwired: 3 in, 5 out]
            n170 = call "_FPGA Set LEDs.vi"("error in (no error)"=w120, "LED Command"=_LED_States."Solid R") -> ()  [unwired: 2 in, 4 out]
          }
          frame 32 {
            w130 = _RT_Instrument_State."24V Standby" ("x")
            w134 = FALSE ("ExhaustGas (on)")
            n171 = global read "_RT Global.vi" "StartupMode"() -> (w128:u8)
            n172 = call "_FPGA Set LEDs.vi"("LED Command"=_LED_States."Solid R") -> ("error out"=w135:errorcluster)  [unwired: 3 in, 3 out]
            n173 = Equal?(x=w130, y=w132) -> (x = y?=w131:bool)
            n174 = Select(t=w130, s=w131, f=w129) -> (s? t:f=w125:T3)
            n175 = Max & Min(x=w128, y=u8 1 ("StartupMode")) -> (max(x,y)=w126:u8)  [unwired: 1 out]
            n176 = global write "_RT Global.vi" "StartupMode"(w126) -> ()
            n177 = call "_FPGA Set Parameters.vi"("ExhaustGas (on)"=w134, "CurGas (on)"=w134, "error in"=w135, "HSID Temp (on)"=w134, "CurInstrState"=w125) -> ()  [unwired: 4 in, 3 out]
          }
          frame 35, 39 {
            n178 = global read "_RT Global.vi" "StartupMode"() -> (w140:u8)
            n179 = call "_FPGA Check Source ID.vi"() -> ("Source ID OK"=w142:bool)  [unwired: 1 in]
            n180 = call "_FPGA Set LEDs.vi"("LED Command"=_LED_States."Solid R") -> ("error out"=w144:errorcluster)  [unwired: 3 in, 3 out]
            n181 = call "_FPGA Set Parameters.vi"("ExhaustGas (on)"=FALSE, "error in"=w144, "HSID Temp (on)"=w142, "CurInstrState"=w137) -> ()  [unwired: 5 in, 3 out]
            n182 = Max & Min(x=w140, y=u8 1 ("StartupMode")) -> (max(x,y)=w138:u8)  [unwired: 1 out]
            n183 = global write "_RT Global.vi" "StartupMode"(w138) -> ()
          }
          frame 40 {
            # "Going to source standby state"
            n184 = global read "_RT Global.vi" "StartupMode"() -> (w150:u8)
            n185 = call "_FPGA Set Parameters.vi"("Source Standby (F)"=TRUE, "HSID Temp (on)"=FALSE, "CurInstrState"=w146) -> ("error out"=w147:errorcluster)  [unwired: 6 in, 2 out]
            n186 = Max & Min(x=w150, y=u8 1 ("StartupMode")) -> (max(x,y)=w148:u8)  [unwired: 1 out]
            n187 = global write "_RT Global.vi" "StartupMode"(w148) -> ()
            n188 = call "_FPGA Set LEDs.vi"("error in (no error)"=w147, "LED Command"=_LED_States."Solid R") -> ()  [unwired: 2 in, 4 out]
          }
        }
        n189 = global write "_RT Global.vi" "ErrorMsg"(w54) -> ()
      }
    }
  }
  "Next InstrState" <- w1
  "Running" <- w5
  n190 = local read "CurInstrState"() -> (w3:T3)
  n191 = Not Equal?(x=w1, y=w3) -> (x != y?=w2:bool)
  n192 = case shown="False" w2 {
    tunnel: w1 -> [_ w386]
    frame False {
    }
    frame True {
      n193 = case shown="\"Lost Communication\"" w386 {
        frame "Initializing", Default {
        }
        frame "Turbopump Ready" {
          n194 = call "_RT Event.vi"("Event"="Going to Turbopump Ready state.") -> ()  [unwired: 2 in, 5 out]
        }
        frame "Lost Communication" {
          n195 = call "_RT Event.vi"("Event"="Going to Lost Communication state.") -> ()  [unwired: 2 in, 5 out]
        }
        frame "Turbopump Ready-Waiting" {
          n196 = call "_RT Event.vi"("Event"="Going to Turbopump Ready-Waiting state.") -> ()  [unwired: 2 in, 5 out]
        }
        frame "Source Standby" {
          n197 = call "_RT Event.vi"("Event"="Going to Source Standby state.") -> ()  [unwired: 2 in, 5 out]
        }
      }
    }
  }
